vi "LVClass_Image Write Image.vi"(8 "error in (no error)":errorcluster, 10 "Image":T1, 11 "Image in":refnum<class "Image.lvclass">) -> (0 "error out":errorcluster, 3 "Image out":refnum<class "Image.lvclass">)   [LabVIEW 2020, in "Image.lvclass"]
uses:
  Image.lvclass
  Struct_Image.ctl
  ClassID.ctl
  Data alignment enum.ctl
  Point2D.ctl
  Handle creation.ctl
  Image.lvclass/Image.ctl
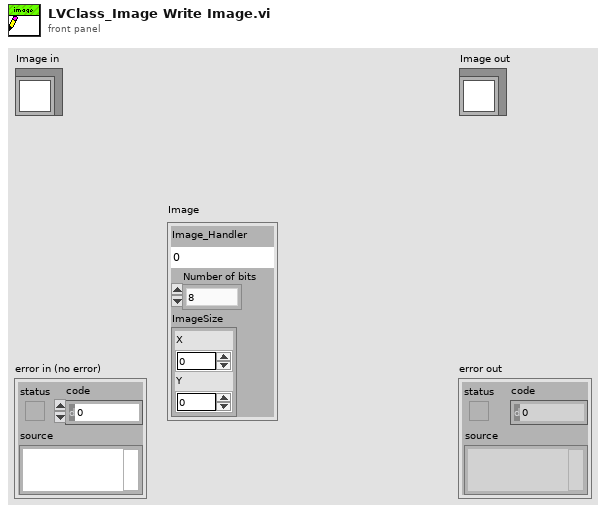
[diagram p1: front panel]
types:
  T1 = typedef "Struct_Image.ctl" = cluster{"Image_Handler":T2, "Number of bits":T3, "ImageSize":T4}
  T2 = typedef "ClassID.ctl" = i64
  T3 = typedef "Data alignment enum.ctl" = enum16{"8", "16", "32"}
  T4 = typedef "Point2D.ctl" = cluster{"X":u32, "Y":u32}
  T5 = typedef "Handle creation.ctl" = enum16{"By ctor", "By write function"}
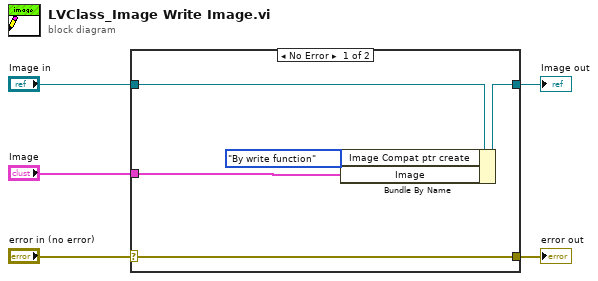
[diagram p0: block diagram]
diagram:
  n1 = case shown="No Error" "error in (no error)" {
    selector: "error in (no error)" -> [w10 w11]
    tunnel: [w10 w11] -> w4
    tunnel: [w8 w12] -> w2
    tunnel: "Image in" -> [w9 w12]
    tunnel: "Image" -> [w7 _]
    frame No Error {
      n2 = Bundle By Name(cluster=w9, "Image Compat ptr create"=Handle_creation."By write function", "Image"=w7) -> (w8:refnum<class "Image.lvclass">)
    }
    frame Error {
    }
  }
  "error out" <- w4
  "Image out" <- w2
